vi "slope2angle.vi"(11 "slope array":dbl[](array[numeric])) -> (0 "rotate angle":dbl, 3 "x/y":dbl[](array[numeric]))   [LabVIEW 2017]
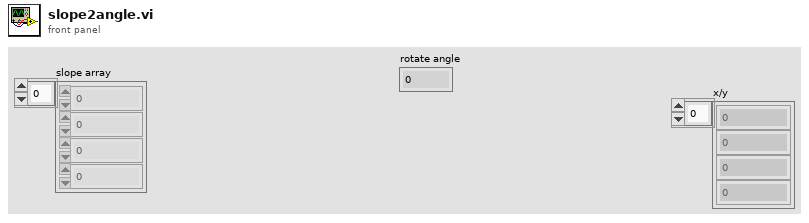
[diagram p1: front panel]
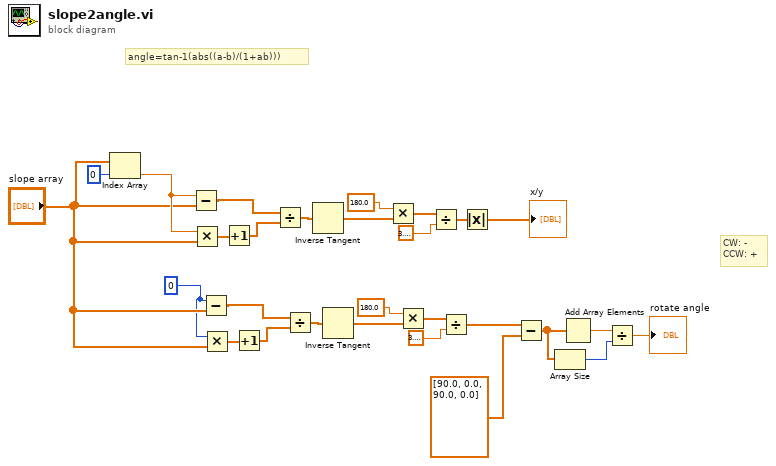
[diagram p0: block diagram]
diagram:
  w7 = 0
  # "CW: -\nCCW: +"
  # "angle=tan-1(abs((a-b)/(1+ab)))"
  n1 = Index Array(array="slope array", index=0) -> (element=w20:dbl)
  n2 = Subtract(x=w20, y="slope array") -> (x-y=w19:dbl[])
  n3 = Multiply(x=w20, y="slope array") -> (x*y=w27:dbl[])
  n4 = Subtract(x=w7, y="slope array") -> (x-y=w16:dbl[])
  n5 = Multiply(x=w7, y="slope array") -> (x*y=w9:dbl[])
  n6 = Increment(x=w27) -> (x+1=w26:dbl[])
  n7 = Increment(x=w9) -> (x+1=w10:dbl[])
  n8 = Divide(x=w19, y=w26) -> (x/y=w25:dbl[])
  n9 = Divide(x=w16, y=w10) -> (x/y=w11:dbl[])
  n10 = Inverse Tangent(1:w25) -> (0:w22:dbl[])
  n11 = Inverse Tangent(1:w11) -> (0:w14:dbl[])
  n12 = Multiply(x=180.0, y=w22) -> (x*y=w21:dbl[])
  n13 = Multiply(x=180.0, y=w14) -> (x*y=w15:dbl[])
  n14 = Divide(x=w21, y=3.141592653589793) -> (x/y=w18:dbl[])
  n15 = Divide(x=w15, y=3.141592653589793) -> (x/y=w5:dbl[])
  n16 = Absolute Value(x=w18) -> (abs(x)=→"x/y":dbl[])
  n17 = Subtract(x=w5, y=dbl[] [90.0, 0.0, 90.0, 0.0] ("x/y")) -> (x-y=w3:dbl[])
  n18 = Array Size(array=w3) -> (size(s)=w2:i32)
  n19 = Add Array Elements(numeric array=w3) -> (sum=w4:dbl)
  n20 = Divide(x=w4, y=w2) -> (x/y=→"rotate angle":dbl)
